vi "Graph-Set.vi"(8 "error in (no error)":errorcluster, 11 "Process in":refnum<vi>) -> (0 "error out":errorcluster, 3 "Data":cluster{dbl, dbl})   [LabVIEW 2016]
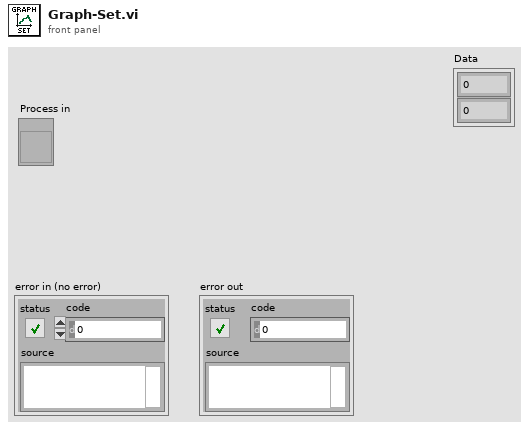
[diagram p1: front panel]
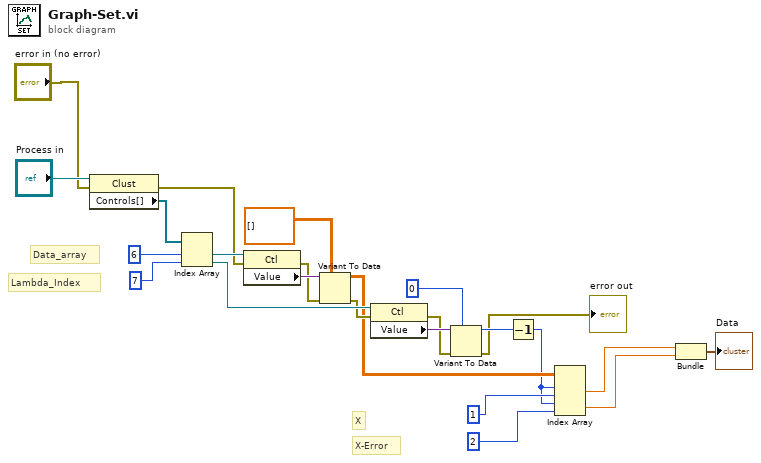
[diagram p0: block diagram]
diagram:
  # "X-Error"
  # "X"
  # "Lambda_Index"
  # "Data_array"
  n1 = property class="Clust"(reference="Process in", error in="error in (no error)") -> (error out=w16:errorcluster, "Controls[]"=w22:refnum<vi>[])  [unwired: 1 out]
  n2 = Index Array(array=w22, index #1=6 ("index"), index #2=7 ("index")) -> (element #1=w19:refnum<vi>, element #2=w14:refnum<vi>)
  n3 = property class="Ctl"(reference=w19, error in=w16) -> (error out=w17:errorcluster, "Value"=w18:variant)  [unwired: 1 out]
  n4 = Variant To Data(error in=w17, type=dbl[][] [], Variant=w18) -> (data=w9:dbl[][], error out=w13:errorcluster)
  n5 = property class="Ctl"(reference=w14, error in=w13) -> (error out=w11:errorcluster, "Value"=w12:variant)  [unwired: 1 out]
  n6 = Variant To Data(error in=w11, type=0, Variant=w12) -> (data=w7:i32, error out=→"error out":errorcluster)
  n7 = Decrement(x=w7) -> (x-1=w6:i32)
  n8 = Index Array(array=w9, index (row) #1=w6, index (col) #1=1 ("disabled index (col)"), index (row) #2=w6, index (col) #2=2 ("disabled index (col)")) -> (element #1=w4:dbl, element #2=w3:dbl)
  n9 = Bundle(w4, w3) -> (→"Data":cluster{dbl, dbl})  [unwired: 1 in]
